vi "Get OBW Results.vi"(8 "error in (no error)":errorcluster, 11 "niDTS BT INSTR TX in":refnum<class "niDTS BT INSTR TX.lvclass">) -> (0 "error out":errorcluster, 2 "OBW Results":T1 {"Stop Frequency (Hz)" format="%#_4p"; "Start Frequency (Hz)" format="%#_4p"}, 3 "niDTS BT INSTR TX out":refnum<class "niDTS BT INSTR TX.lvclass">)   [LabVIEW 2015, in "niDTS BT.lvlib" / "niDTS BT INSTR TX.lvclass"]
uses:
  niDTS BT INSTR TX.lvclass
  Tests/Tx Test/Includes/niDTS BT Tx Test INC OBW Results.ctl
  niDTS BT INSTR TX.lvclass/niDTS BT INSTR TX.ctl
  RiviInstDriver/niRfsaBT/Objects/niRfsaBt.lvclass
  niDTS BT.lvlib
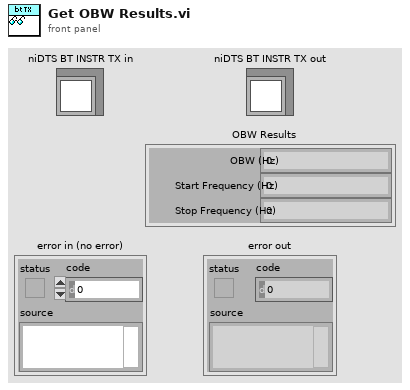
[diagram p1: front panel]
types:
  T1 = typedef "niDTS BT.lvlib/niDTS BT Tx Test INC OBW Results.ctl" = cluster{"OBW (Hz)":dbl, "Start Frequency (Hz)":dbl, "Stop Frequency (Hz)":dbl}
  T2 = cluster{"OccupiedBandwidth":dbl, "StartFrequency":dbl, "StopFrequency":dbl}
  T3 = typedef "niRfsaBT.lvclass/niRfsaBT INC Handle.ctl" = refnum<data-value>
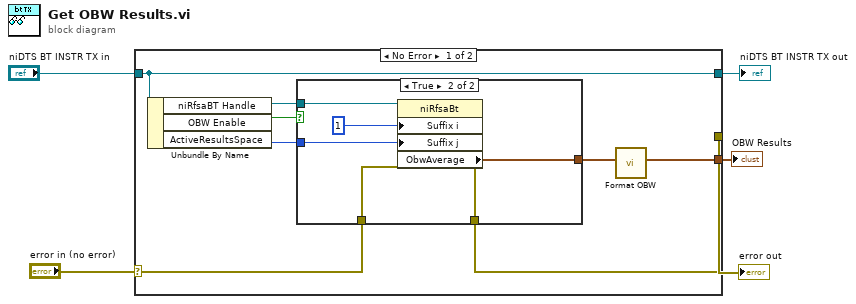
[diagram p0: block diagram]
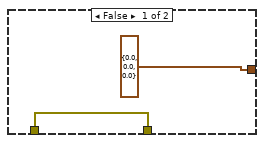
[diagram p2: hidden frame]
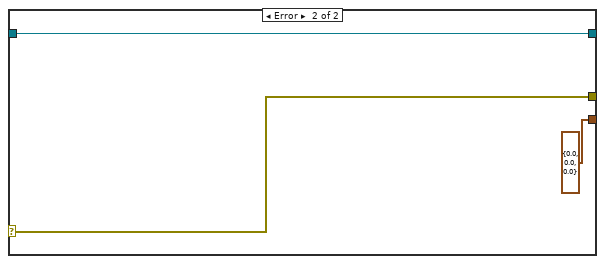
[diagram p3: hidden frame]
diagram:
  n1 = case shown="No Error" "error in (no error)" {
    selector: "error in (no error)" -> [w10 w23]
    tunnel: [w9 w23] -> w4
    tunnel: [w11 w24] -> w2
    tunnel: "niDTS BT INSTR TX in" -> [w11 w24]
    tunnel: [w7 T1 {"OBW (Hz)"=0.0, "Start Frequency (Hz)"=0.0, "Stop Frequency (Hz)"=0.0} ("OBW Results")] -> w1
    frame No Error {
      n2 = Unbundle By Name(w11) -> ("niRfsaBT Handle"=w13:T3, "OBW Enable"=w12:bool, "ActiveResultsSpace"=w6:u8)
      n3 = case shown="True" w12 {
        tunnel: w13 -> [_ w21]
        tunnel: w10 -> [w14 w17]
        tunnel: [w14 w20] -> w9
        tunnel: [T2 {"OccupiedBandwidth"=0.0, "StartFrequency"=0.0, "StopFrequency"=0.0} ("[SPAN]") w18] -> w8
        tunnel: w6 -> [_ w16]
        frame False {
        }
        frame True {
          n4 = property class="niRfsaBt"(reference=w21, error in=w17, "Suffix i"=1 ("Active Channel:Suffix i"), "Suffix j"=w16) -> (error out=w20:errorcluster, "ObwAverage"=w18:T2)  [unwired: 1 out]
        }
      }
      n5 = call "Format OBW.vi"("OBW"=w8) -> ("OBW Results"=w7:T1)  [unwired: 10 in]
    }
    frame Error {
    }
  }
  "error out" <- w4
  "niDTS BT INSTR TX out" <- w2
  "OBW Results" <- w1
